vi "OPC UA Client-Read with Subscription.vi"() -> ()   [LabVIEW 2017]
uses:
  <vilib>/OPCUA/NI OPC UA Client.lvlib
panel:
  out "Time Stamp":timestamp=timestamp(3500457874.2072477 s since 1904-01-01) format="%<%Y.%m.%d %H:%M:%S>T"
  in  "Item Path":string="Process Data.Temperature"
  in  "Stop Button":bool
  out "Temperature Value":dbl=8.0
  in  "Server Endpoint URL":string="opc.tcp://XPS15HPH:49580"
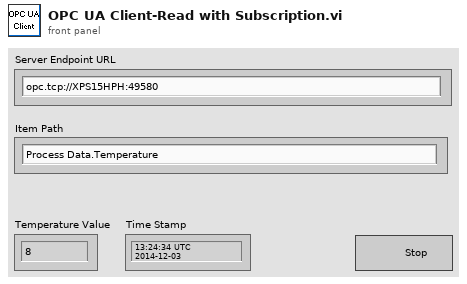
[diagram p1: front panel]
types:
  T1 = cluster{"message mode":enum16{"None", "Sign", "Sign and Encrypt"}, "security":enum16{"Basic256", "Basic128Rsa15"}}
  T2 = typedef "OPC UA Client Refnum.ctl" = refnum<k21>
  T3 = typedef "Subscription ID.ctl" = u32
  T4 = typedef "Subscription Data Change.ctl" = cluster{"node ID":T5, " value":variant, "timestamp":timestamp, "data type":T6, "status code":T7}
  T5 = typedef "NodeId.ctl" = string
  T6 = typedef "Data Type.ctl" = u16
  T7 = typedef "OPC UA StatusCode.ctl" = u32
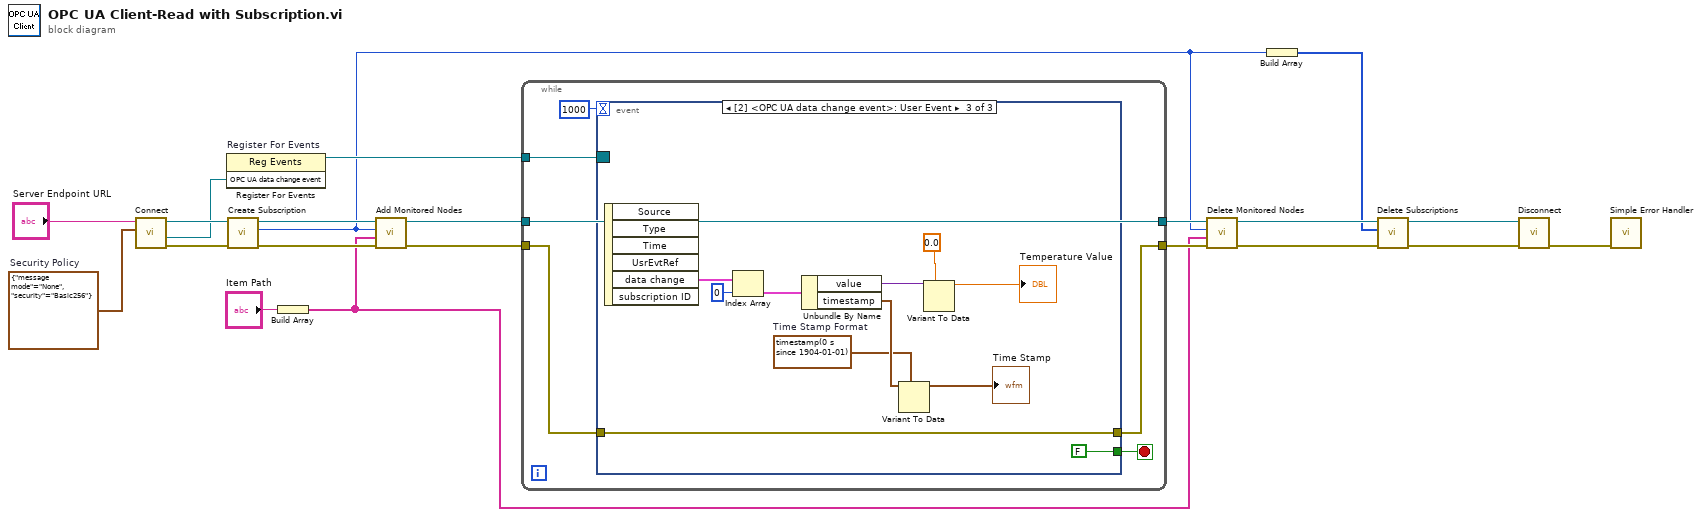
[diagram p0: block diagram]
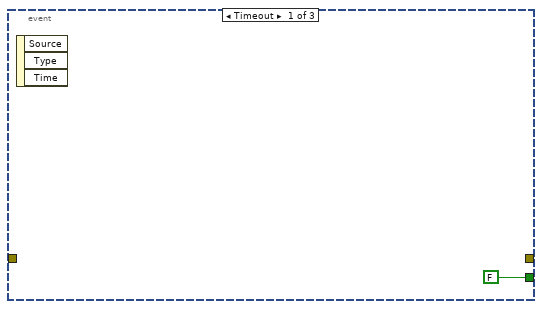
[diagram p2: hidden frame]
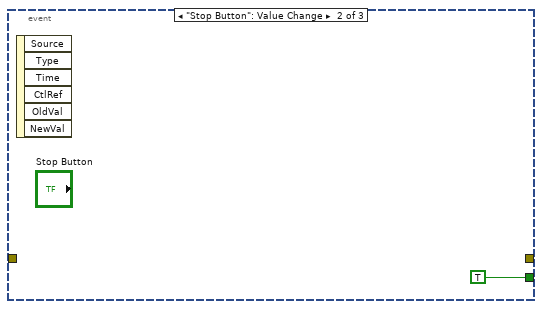
[diagram p3: hidden frame]
diagram:
  w19 = T1 {"message mode"=enum."None", "security"=enum."Basic256"}  # Security Policy
  n1 = call <vilib>:"Connect.vi"("security policy"=w19, "server endpoint URL"="Server Endpoint URL") -> ("error out"=w9:errorcluster, "OPC UA data change event"=w6:refnum<user-event>, "OPC UA client refnum out"=w12:T2)  [unwired: 7 in]
  n2 = register-events "Register For Events"(w6) -> (reference out=w5:refnum<event-registration>)  [unwired: 2 in, 1 out]
  n3 = call <vilib>:"Create Subscription.vi"("error in (no error)"=w9, "OPC UA client refnum in"=w12) -> ("error out"=w10:errorcluster, "subscription ID out"=w1:T3, "OPC UA client refnum out"=w11:T2)  [unwired: 5 in, 2 out]
  n4 = Build Array "Build Array"("Item Path") -> (w3:string[])
  n5 = call <vilib>:"Add Monitored Nodes.vi"("error in (no error)"=w10, "node IDs"=w3, "subscription ID in"=w1, "OPC UA client refnum in"=w11) -> ("error out"=w7:errorcluster, "OPC UA client refnum out"=w8:T2)  [unwired: 5 in, 1 out]
  n6 = while {
    tunnel: w8 -> [w26]
    tunnel: w7 -> [w23]
    tunnel: [w26] -> w15
    tunnel: [w22] -> w18
    tunnel: w5 -> [w27]
    stop <- w24 stop-if-true
    n7 = event shown="[2] <OPC UA data change event>: User Event" {
      selector: w27 -> [_ _ _]
      dyn-events: _ -> [_ _ _]
      timeout: 1000 -> [_ _ _]
      tunnel: [FALSE TRUE FALSE] -> w24
      tunnel: w23 -> [_ _ w39]
      tunnel: [_ _ w39] -> w22
      event Timeout {
        n8 = event-data() -> ()  [unwired: 1 in, 3 out]
      }
      event "Stop Button": Value Change {
        n9 = event-data() -> ()  [unwired: 1 in, 6 out]
      }
      event User Event {
        w31 = timestamp(0 s since 1904-01-01)  # Time Stamp Format
        n10 = event-data() -> ("data change"=w38:T4[])  [unwired: 1 in, 5 out]
        n11 = Index Array "Index Array"(array=w38, index=0) -> (element=w36:T4)
        n12 = Unbundle By Name "Unbundle By Name"(w36) -> ("value"=w35:variant, "timestamp"=w32:timestamp)
        n13 = Variant To Data(type=w31, Variant=w32) -> (data=→"Time Stamp":timestamp)  [unwired: 1 in, 1 out]
        n14 = Variant To Data(type=0.0 ("Temperature Value"), Variant=w35) -> (data=→"Temperature Value":dbl)  [unwired: 1 in, 1 out]
      }
    }
  }
  n15 = call <vilib>:"Delete Monitored Nodes.vi"("error in (no error)"=w18, "node IDs"=w3, "subscription ID in"=w1, "OPC UA client refnum in"=w15) -> ("error out"=w17:errorcluster, "OPC UA client refnum out"=w14:T2)  [unwired: 3 in, 3 out]
  n16 = Build Array "Build Array"(w1) -> (w2:T3[])
  n17 = call <vilib>:"Delete Subscriptions.vi"("error in (no error)"=w17, "subscription IDs"=w2, "OPC UA client refnum in"=w14) -> ("error out"=w16:errorcluster, "OPC UA client refnum out"=w13:T2)  [unwired: 6 in, 1 out]
  n18 = call <vilib>:"Disconnect.vi"("error in (no error)"=w16, "OPC UA client refnum in"=w13) -> ("error out"=w21:errorcluster)  [unwired: 9 in]
  n19 = call <vilib>:"Simple Error Handler.vi"("error in (no error)"=w21) -> ()  [unwired: 4 in, 5 out]
